vi "set_trigger.vi"(8 "error in (no error)":errorcluster, 9 "edge":T1, 10 "digital trigger line":tag, 11 "DAQmxWriteSignals in":refnum<class "SignalWriterMM140725DAQmx.lvclass">) -> (0 "error out":errorcluster, 3 "DAQmxWriteSignals out":refnum<class "SignalWriterMM140725DAQmx.lvclass">)   [LabVIEW 2010, in "SignalWriterMM140725DAQmx.lvclass"]
uses:
  SignalWriterMM140725DAQmx.lvclass
  trigger_edge_enum.ctl
  SignalWriterMM140725DAQmx.lvclass/SignalWriterMM140725DAQmx.ctl
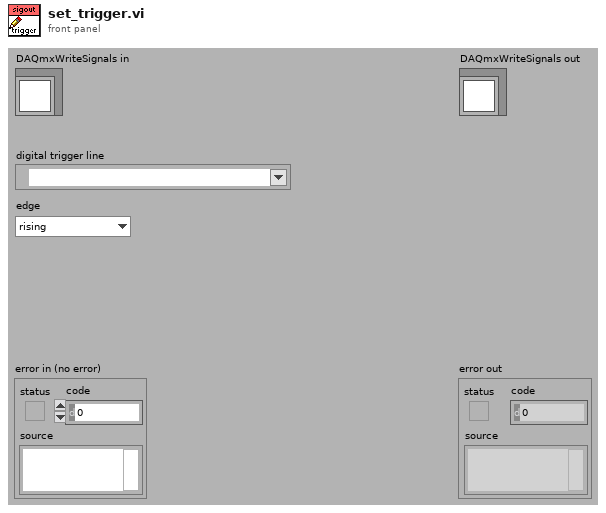
[diagram p1: front panel]
types:
  T1 = typedef "SignalWriterMM140725DAQmx.lvclass/trigger_edge_enum.ctl" = enum16{"rising", "falling"}
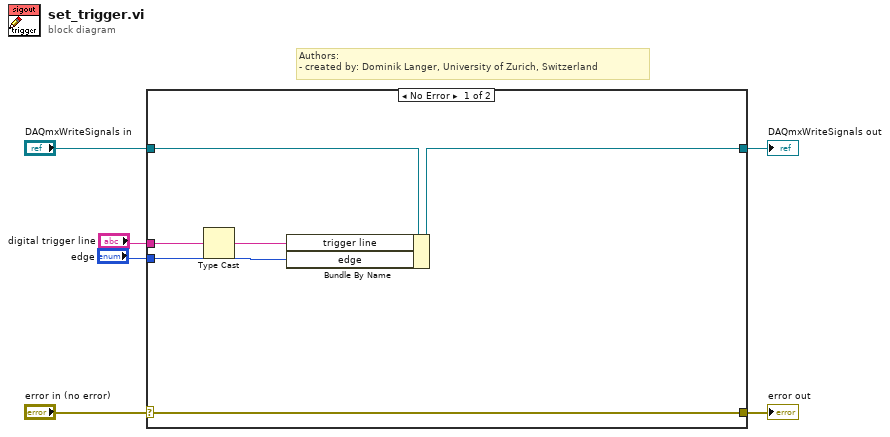
[diagram p0: block diagram]
diagram:
  # "Authors: \n- created by: Dominik Langer, University of Zurich, Switzerland"
  n1 = case shown="No Error" "error in (no error)" {
    selector: "error in (no error)" -> [w12 w14]
    tunnel: [w12 w14] -> w5
    tunnel: [w7 w13] -> w3
    tunnel: "DAQmxWriteSignals in" -> [w8 w13]
    tunnel: "edge" -> [w11 _]
    tunnel: "digital trigger line" -> [w9 _]
    frame No Error {
      n2 = Type Cast(x=w9) -> (*(type *) &x=w10:string)  [unwired: 1 out]
      n3 = Bundle By Name(cluster=w8, "trigger line"=w10, "edge"=w11) -> (w7:refnum<class "SignalWriterMM140725DAQmx.lvclass">)
    }
    frame Error {
    }
  }
  "error out" <- w5
  "DAQmxWriteSignals out" <- w3
